vi "11_Histogram2D.vi"(8 "error in (no error)":errorcluster) -> (0 "error out":errorcluster)   [LabVIEW 2014]
uses:
  SwabianInstruments.TimeTagger
panel:
  in  "binwidth":i64=1
  in  "n_bins_2":i32=300
  in  "n_bins_1":i32=400
  out "Histogram2D":i32[][](graph)
  # "Histogram2D. Each pixel represent a bin with the bin value as color.\nEach bin corresponds to specific time delay between each stop signal and the start signal.\nSo the bin coordinate to de incremented is calculated as (stop1-start, stop2-start) rounded to \nthe corersponding bin boundary.\n\nIn this example we use internal signal generator as start, stop1 and stop2 signals we expect to see \na small, jitter limited, Gaussian like spot located at the position that is generally offset from zero due to small delay \ndifference between channels."
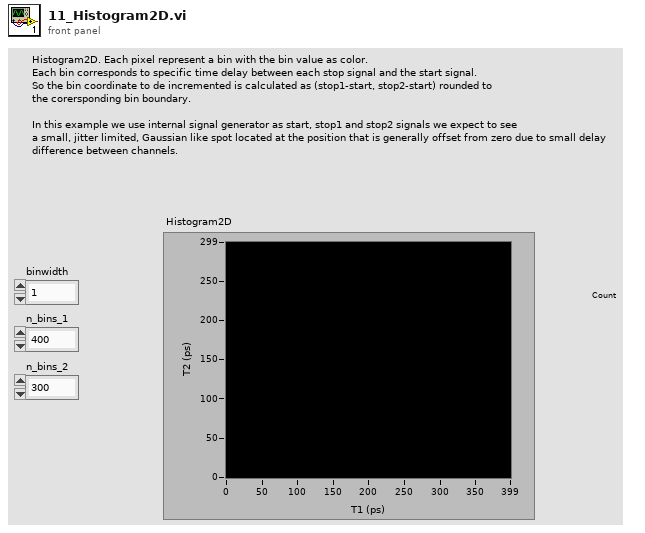
[diagram p1: front panel]
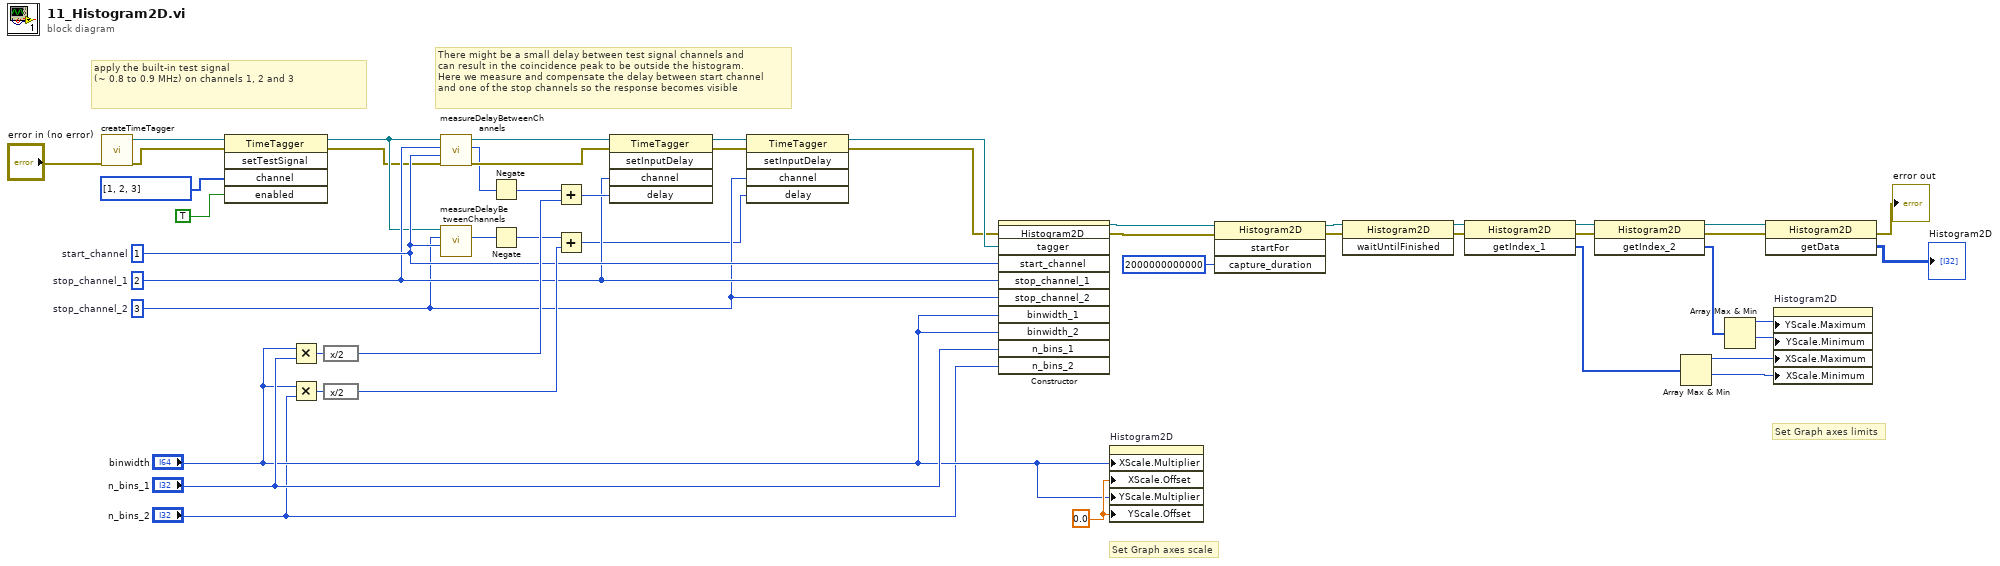
[diagram p0: block diagram]
diagram:
  w42 = 0.0 ("X Scale.Offset and Multiplier:Offset")
  w15 = 3  # stop_channel_2
  w16 = 2  # stop_channel_1
  w17 = 1  # start_channel
  # "There might be a small delay between test signal channels and \ncan result in the coincidence peak to be outside the histogram.\nHere we measure and compensate the delay between start channel\nand one of the stop channels so the response becomes visible"
  # "Set Graph axes limits"
  # "Set Graph axes scale"
  # "apply the built-in test signal\n(~ 0.8 to 0.9 MHz) on channels 1, 2 and 3"
  n1 = call "createTimeTagger.vi"("error in (no error)"="error in (no error)") -> ("error out"=w34:errorcluster, "TimeTagger ref out"=w35:refnum<k24>)  [unwired: 9 in]
  n2 = invoke class="TimeTagger" method="setTestSignal"(reference=w35, error in=w34, "channel"=i32[] [1, 2, 3], "enabled"=TRUE) -> (reference out=w13:refnum<k24>, error out=w12:errorcluster)  [unwired: 1 in, 3 out]
  n3 = Multiply(x="binwidth", y="n_bins_1") -> (x*y=w26:i64)
  n4 = Multiply(x="binwidth", y="n_bins_2") -> (x*y=w25:i64)
  n5 = expression code="x/2"(w26) -> (w24:i64)
  n6 = expression code="x/2"(w25) -> (w23:i64)
  n7 = call "measureDelayBetweenChannels.vi"("error in (no error)"=w12, "channel_2"=w17, "channel_1"=w16, "TimeTagger ref in"=w13) -> ("error out"=w32:errorcluster, "measured delay, ps"=w31:i64, "TimeTagger ref out"=w33:refnum<k24>)  [unwired: 5 in]
  n8 = call "measureDelayBetweenChannels.vi"("channel_2"=w17, "channel_1"=w15, "TimeTagger ref in"=w13) -> ("measured delay, ps"=w21:i64)  [unwired: 6 in, 2 out]
  n9 = Negate(x=w31) -> (-x=w30:i64)
  n10 = Negate(x=w21) -> (-x=w20:i64)
  n11 = Add(x=w30, y=w24) -> (x+y=w22:i64)
  n12 = Add(x=w20, y=w23) -> (x+y=w14:i64)
  n13 = invoke class="TimeTagger" method="setInputDelay"(reference=w33, error in=w32, "channel"=w16, "delay"=w22) -> (reference out=w19:refnum<k24>, error out=w18:errorcluster)  [unwired: 1 in, 3 out]
  n14 = invoke class="TimeTagger" method="setInputDelay"(reference=w19, error in=w18, "channel"=w15, "delay"=w14) -> (reference out=w11:refnum<k24>, error out=w10:errorcluster)  [unwired: 1 in, 3 out]
  n15 = constructor class="Histogram2D"(error in=w10, "tagger"=w11, "start_channel"=w17, "stop_channel_1"=w16, "stop_channel_2"=w15, "binwidth_1"="binwidth", "binwidth_2"="binwidth", "n_bins_1"="n_bins_1", "n_bins_2"="n_bins_2") -> (reference out=w9:refnum<k24>, error out=w8:errorcluster)  [unwired: 2 in, 9 out]
  n16 = property on="Histogram2D" class="IntGraph (strict)"("XScale.Multiplier"="binwidth", "XScale.Offset"=w42, "YScale.Multiplier"="binwidth", "YScale.Offset"=w42) -> ()  [unwired: 2 in, 2 out]
  n17 = invoke class="Histogram2D" method="startFor"(reference=w9, error in=w8, "capture_duration"=i64 2000000000000) -> (reference out=w6:refnum<k24>, error out=w3:errorcluster)  [unwired: 1 in, 2 out]
  n18 = invoke class="Histogram2D" method="waitUntilFinished"(reference=w6, error in=w3) -> (reference out=w5:refnum<k24>, error out=w4:errorcluster)  [unwired: 1 in, 1 out]
  n19 = invoke class="Histogram2D" method="getIndex_1"(reference=w5, error in=w4) -> (reference out=w46:refnum<k24>, error out=w45:errorcluster, "getIndex_1"=w41:i64[])  [unwired: 1 in]
  n20 = invoke class="Histogram2D" method="getIndex_2"(reference=w46, error in=w45) -> (reference out=w43:refnum<k24>, error out=w44:errorcluster, "getIndex_2"=w40:i64[])  [unwired: 1 in]
  n21 = Array Max & Min(array=w41) -> (max value=w37:i64, min value=w36:i64)  [unwired: 2 out]
  n22 = Array Max & Min(array=w40) -> (max value=w39:i64, min value=w38:i64)  [unwired: 2 out]
  n23 = invoke class="Histogram2D" method="getData"(reference=w43, error in=w44) -> (error out=→"error out":errorcluster, "getData"=→"Histogram2D":i32[][])  [unwired: 1 in, 1 out]
  n24 = property on="Histogram2D" class="IntGraph (strict)"("YScale.Maximum"=w39, "YScale.Minimum"=w38, "XScale.Maximum"=w37, "XScale.Minimum"=w36) -> ()  [unwired: 2 in, 2 out]
